vi "Dispersion.vi"() -> ()   [LabVIEW 2010]
uses:
  pulse parameters.ctl
  toolbar icons/log data.ctl
  toolbar icons/Open calibration.ctl
  toolbar icons/Save calibration.ctl
  ADT 2/help.ctl
  file/file action.ctl
panel:
  in  "Help Button":T1
  in  "Save Method":T2
  in  "Open Method":T3
  out "signal array":dbl[][](array[numeric])
  in  "Save Data":T4
  out "F pulse train graph":cluster{dbl[], dbl[]}[](graph)
  in  "pulse parameters":T5={"Pe"=400.0, "dt"=0.001, "duty"=0.44999999999999996, "cycle time"=0.2, "Integration error"=0.0001, "cycles"=4} {"cycles" min=1; "cycle time" min=0.0; "duty" min=0.0 max=1.0; "dt" min=1e-12; "Pe" min=0.0}
  out "E pulse graph":cluster{"t*":dbl[], dbl[]}(graph)
  in  "stop":bool
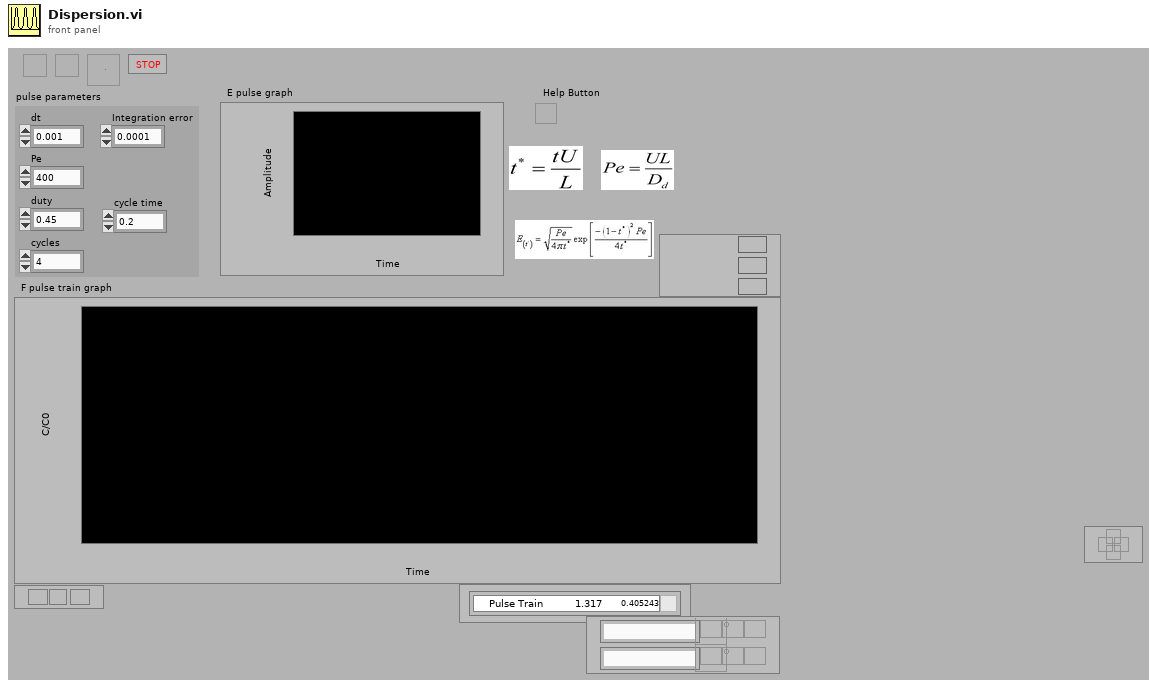
[diagram p1: front panel]
types:
  T1 = typedef "help.ctl" = bool
  T2 = typedef "Save calibration.ctl" = bool
  T3 = typedef "Open calibration.ctl" = bool
  T4 = typedef "log data.ctl" = bool
  T5 = typedef "pulse parameters.ctl" = cluster{"Pe":dbl, "dt":dbl, "duty":dbl, "cycle time":dbl, "Integration error":dbl, "cycles":i16}
  T6 = typedef "file action.ctl" = enum16{"Save", "Open"}
  T7 = cluster{"t* pulse train":dbl[], "input waveform":dbl[]}
  T8 = cluster{"Ramp Pattern":dbl[], "input waveform":dbl[]}[]
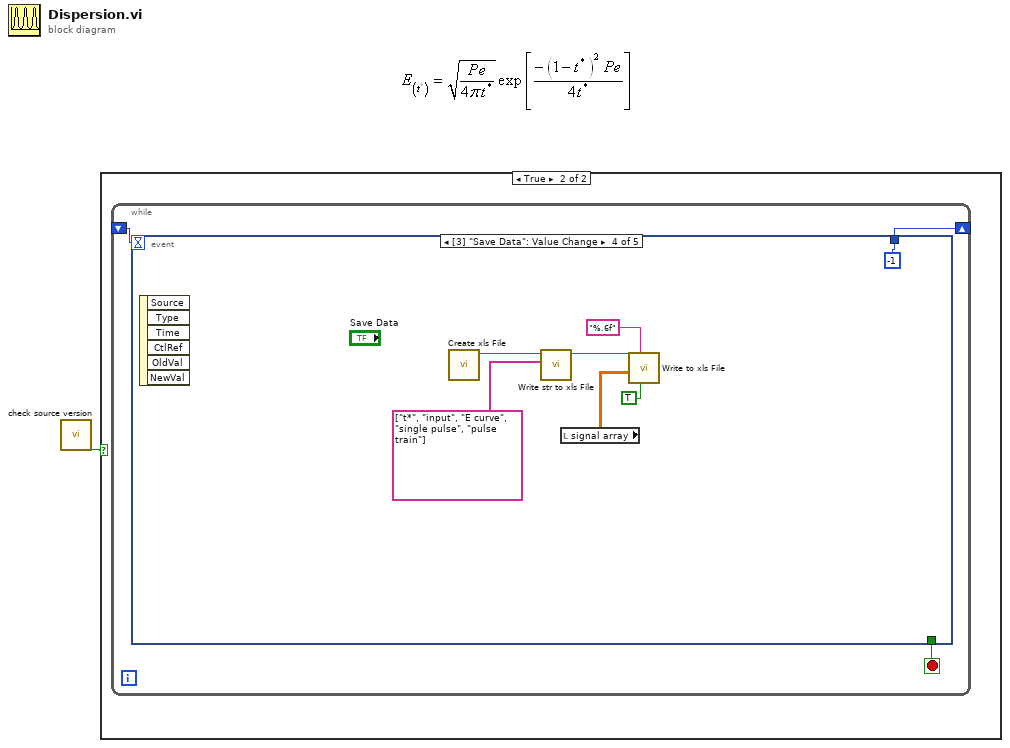
[diagram p0: block diagram]
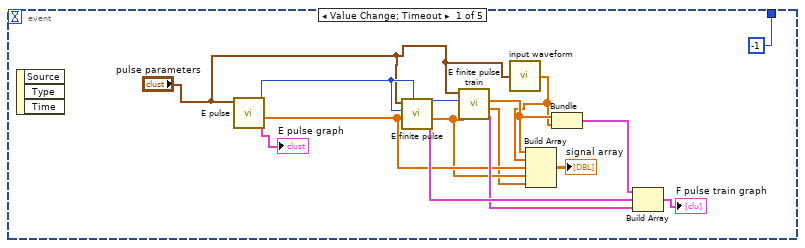
[diagram p3: hidden frame]
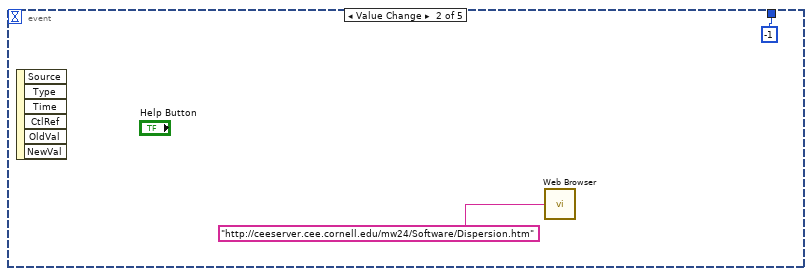
[diagram p4: hidden frame]
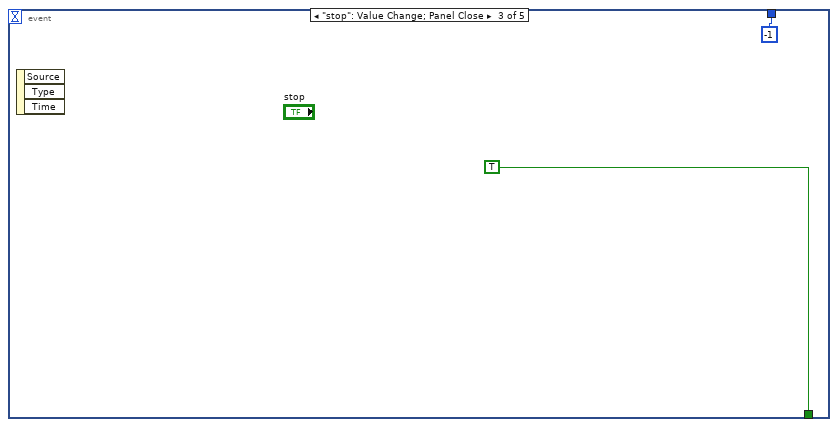
[diagram p5: hidden frame]
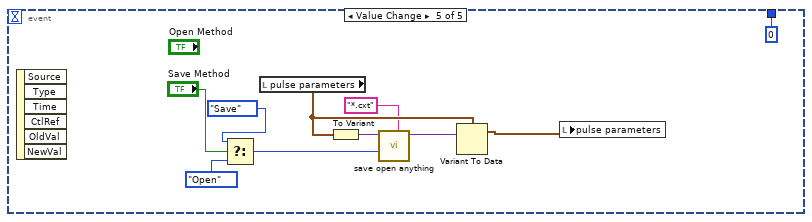
[diagram p6: hidden frame]
diagram:
  n1 = call "check source version.vi"() -> ("continue running?"=w1:bool)  [unwired: 2 in, 3 out]
  n2 = case shown="True" w1 {
    frame False {
    }
    frame True {
      n3 = while {
        shift-right: [w2] -> _
        shift-left: _ -> [w3]
        stop <- w4 stop-if-true
        n4 = event shown="[3] \"Save Data\": Value Change" {
          selector: _ -> [_ _ _ _ _]
          dyn-events: _ -> [_ _ _ _ _]
          timeout: w3 -> [_ _ _ _ _]
          tunnel: [_ _ TRUE _ _] -> w4
          tunnel: [-1 -1 -1 -1 0] -> w2
          event Value Change; Timeout {
            n5 = event-data() -> ()  [unwired: 1 in, 3 out]
            n6 = call "E pulse.vi"("pulse parameters"="pulse parameters") -> ("E graph"=→"E pulse graph":cluster{"t*":dbl[], dbl[]}, "E"=w9:dbl[], "t*/theta"=w18:i16)  [unwired: 7 in, 1 out]
            n7 = call "E finite pulse.vi"("E"=w9, "t*/theta"=w18, "pulse parameters"="pulse parameters") -> ("F finite graph"=w16:cluster{"t*":dbl[], dbl[]}, "F finite"=w8:dbl[])  [unwired: 6 in, 1 out]
            n8 = call "E finite pulse train.vi"("F finite"=w8, "t*/theta"=w18, "pulse parameters"="pulse parameters") -> ("F pulse train graph"=w15:cluster{"Ramp Pattern":dbl[], dbl[]}, "F pulse train"=w7:dbl[], "t* pulse train"=w11:dbl[])  [unwired: 6 in]
            n9 = call "input waveform.vi"("pulse parameters"="pulse parameters") -> ("input waveform"=w10:dbl[])
            n10 = Build Array(w11, w10, w9, w8, w7) -> (→"signal array":dbl[][])
            n11 = Bundle("t* pulse train"=w11, "input waveform"=w10) -> (w12:T7)  [unwired: 1 in]
            n12 = Build Array(w12, w16, w15) -> (→"F pulse train graph":T8)
          }
          event Value Change {
            n13 = event-data() -> ()  [unwired: 1 in, 6 out]
            n14 = call "Web Browser.vi"("URL"="http://ceeserver.cee.cornell.edu/mw24/Software/Dispersion.htm") -> ()  [unwired: 1 in]
          }
          event "stop": Value Change; Panel Close {
            n15 = event-data() -> ()  [unwired: 1 in, 3 out]
          }
          event Value Change {
            n16 = event-data() -> ()  [unwired: 1 in, 6 out]
            n17 = call "Create xls File.vi"() -> ("refnum"=w29:refnum<file>)  [unwired: 4 in, 3 out]
            n18 = call "Write str to xls File.vi"("1D data"=string[] ["t*", "input", "E curve", "single pulse", "pulse train"], "refnum"=w29) -> ("dup refnum"=w28:refnum<file>)  [unwired: 8 in, 1 out]
            n19 = local read "signal array"() -> (w26:dbl[][])
            n20 = call "Write to xls File.vi"("transpose? (no:F)"=TRUE, "format (%.3f)"="%.6f", "2D data"=w26, "refnum"=w28) -> ()  [unwired: 6 in, 2 out]
          }
          event Value Change {
            n21 = event-data() -> ()  [unwired: 1 in, 6 out]
            n22 = Select(t=file_action."Save" ("Action"), s="Save Method", f=file_action."Open" ("Action")) -> (s? t:f=w36:T6)
            n23 = local read "pulse parameters"() -> (w33:T5)
            n24 = To Variant(anything=w33) -> (Variant=w39:variant)
            n25 = call "save open anything.vi"("Variant"=w39, "Action"=w36, "pattern"="*.cxt") -> ("Variant out"=w34:variant)  [unwired: 4 in, 3 out]
            n26 = Variant To Data(Variant=w34, type=w33) -> (data=w32:T5)  [unwired: 1 in, 1 out]
            n27 = local write "pulse parameters"(w32) -> ()
          }
        }
      }
    }
  }
